vi "CloseScope.vi"(8 "error in":errorcluster, 11 "Acquisition Unit in (0)":i32) -> (0 "error out":errorcluster, 3 "Acquisition Unit out":i32, 4 "CAU status":T1)   [LabVIEW 2009]
uses:
  libraries/Cscope control driver.llb/Cscope intf status.ctl
  libraries/Cscope control driver.llb/Cscope control command type.ctl
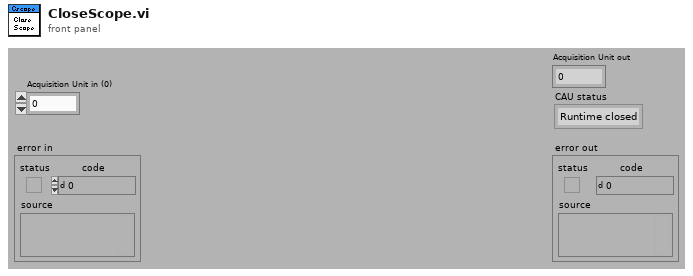
[diagram p1: front panel]
types:
  T1 = typedef "Cscope intf status.ctl" = enum16{"Runtime closed", "Closed", "Open", "Fault", "Fault closed"}
  T2 = typedef "Cscope control command type.ctl" = enum16{"Initialize", "Acquire", "Replay", "Wait for samples", "Update", "Close", "Status", "Function", "Get Frame", "Finish", "Function Result", "Check Got Samples", "Get Chan A", "Get Chan B", "Get Dig"}
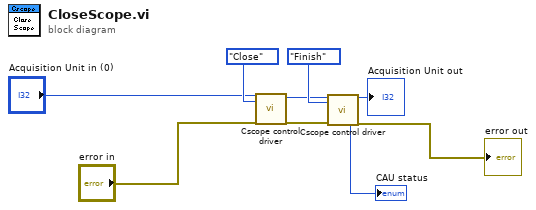
[diagram p0: block diagram]
diagram:
  n1 = call "Cscope control driver.vi"("Acquisition Unit in"="Acquisition Unit in (0)", "Command"=Cscope_control_command_type."Close", "error in"="error in") -> ("Acquisition Unit out"=w2:i32, "error out"=w7:errorcluster)  [unwired: 5 in, 10 out]
  n2 = call "Cscope control driver.vi"("Acquisition Unit in"=w2, "Command"=Cscope_control_command_type."Finish", "error in"=w7) -> ("CAU status"=→"CAU status":T1, "Acquisition Unit out"=→"Acquisition Unit out":i32, "error out"=→"error out":errorcluster)  [unwired: 5 in, 9 out]
